vi "template-lstm-cell.vi"(7 "x":T1, 9 "h":T1, 11 "c":T1) -> (1 "h + 1":T1, 3 "c + 1":T1)   [LabVIEW 2020]
uses:
  <vilib>/Analysis/Matrix/Datatypes/RealMatrix.ctl
  <vilib>/Analysis/Matrix/Numeric/Multiply/Multiply - RM,RM.vi
  <vilib>/Analysis/Matrix/Numeric/Add/Add - RM,RM.vi
  <vilib>/Analysis/Matrix/NI_Matrix.lvlib
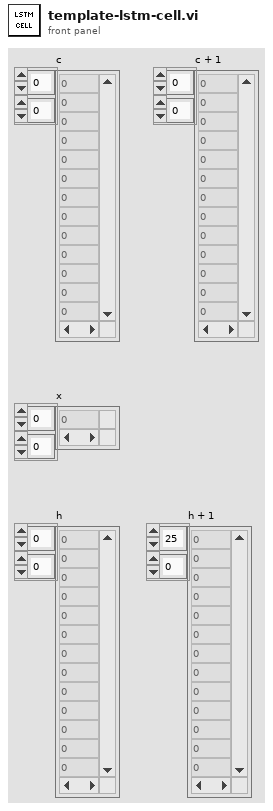
[diagram p1: front panel]
types:
  T1 = typedef "NI_Matrix.lvlib/RealMatrix.ctl" = dbl[][]
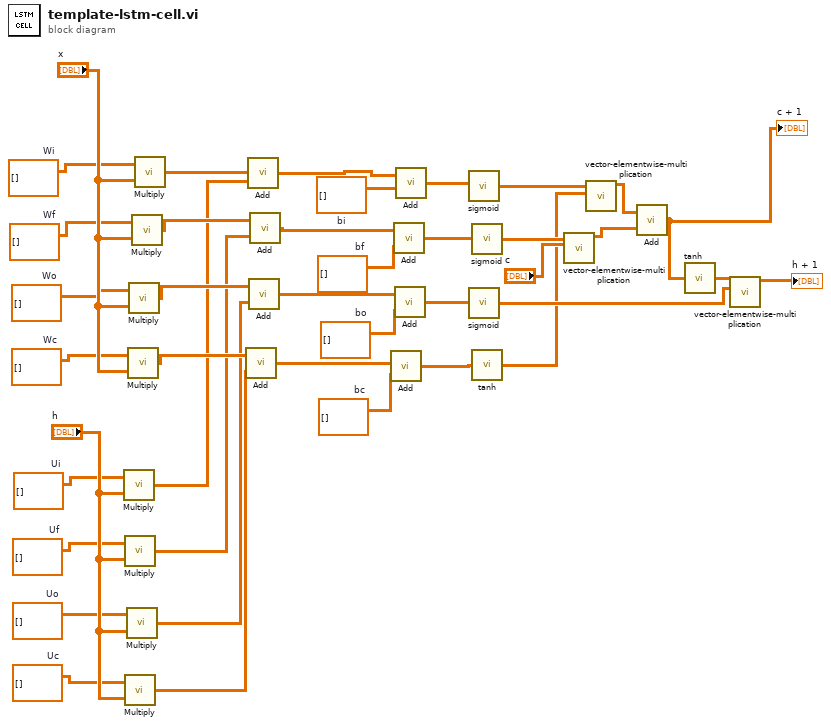
[diagram p0: block diagram]
diagram:
  w31 = T1 []  # Uo
  w17 = T1 []  # bo
  w38 = T1 []  # Wf
  w33 = T1 []  # Uf
  w37 = T1 []  # Wo
  w21 = T1 []  # bi
  w34 = T1 []  # Ui
  w39 = T1 []  # Wi
  w15 = T1 []  # bc
  w32 = T1 []  # Uc
  w36 = T1 []  # Wc
  w19 = T1 []  # bf
  n1 = call-poly <vilib>:"Multiply.vi"("Real Matrix B"="h", "Real Matrix A"=w34) -> ("A * B"=w26:T1)
  n2 = call-poly <vilib>:"Multiply.vi"("Real Matrix B"="h", "Real Matrix A"=w33) -> ("A * B"=w25:T1)
  n3 = call-poly <vilib>:"Multiply.vi"("Real Matrix B"="h", "Real Matrix A"=w32) -> ("A * B"=w23:T1)
  n4 = call-poly <vilib>:"Multiply.vi"("Real Matrix B"="h", "Real Matrix A"=w31) -> ("A * B"=w24:T1)
  n5 = call-poly <vilib>:"Multiply.vi"("Real Matrix B"="x", "Real Matrix A"=w36) -> ("A * B"=w27:T1)
  n6 = call-poly <vilib>:"Multiply.vi"("Real Matrix B"="x", "Real Matrix A"=w37) -> ("A * B"=w28:T1)
  n7 = call-poly <vilib>:"Multiply.vi"("Real Matrix B"="x", "Real Matrix A"=w38) -> ("A * B"=w29:T1)
  n8 = call-poly <vilib>:"Multiply.vi"("Real Matrix B"="x", "Real Matrix A"=w39) -> ("A * B"=w30:T1)
  n9 = call-poly <vilib>:"Add.vi"("Real Matrix B"=w23, "Real Matrix A"=w27) -> ("A + B"=w16:T1)
  n10 = call-poly <vilib>:"Add.vi"("Real Matrix B"=w26, "Real Matrix A"=w30) -> ("A + B"=w22:T1)
  n11 = call-poly <vilib>:"Add.vi"("Real Matrix B"=w24, "Real Matrix A"=w28) -> ("A + B"=w18:T1)
  n12 = call-poly <vilib>:"Add.vi"("Real Matrix B"=w25, "Real Matrix A"=w29) -> ("A + B"=w20:T1)
  n13 = call-poly <vilib>:"Add.vi"("Real Matrix B"=w15, "Real Matrix A"=w16) -> ("A + B"=w10:T1)
  n14 = call-poly <vilib>:"Add.vi"("Real Matrix B"=w19, "Real Matrix A"=w20) -> ("A + B"=w13:T1)
  n15 = call-poly <vilib>:"Add.vi"("Real Matrix B"=w17, "Real Matrix A"=w18) -> ("A + B"=w12:T1)
  n16 = call-poly <vilib>:"Add.vi"("Real Matrix B"=w21, "Real Matrix A"=w22) -> ("A + B"=w14:T1)
  n17 = call "sigmoid.vi"("x"=w14) -> ("y"=w4:T1)
  n18 = call "sigmoid.vi"("x"=w12) -> ("y"=w7:T1)
  n19 = call "sigmoid.vi"("x"=w13) -> ("y"=w9:T1)
  n20 = call "tanh.vi"("x"=w10) -> ("y"=w5:T1)
  n21 = call "vector-elementwise-multiplication.vi"("Matrix in"="c", "Matrix 1"=w9) -> ("elementwise product"=w2:T1)  [unwired: 9 in]
  n22 = call "vector-elementwise-multiplication.vi"("Matrix in"=w5, "Matrix 1"=w4) -> ("elementwise product"=w3:T1)  [unwired: 9 in]
  n23 = call-poly <vilib>:"Add.vi"("Real Matrix B"=w2, "Real Matrix A"=w3) -> ("A + B"=w1:T1)
  "c + 1" <- w1
  n24 = call "tanh.vi"("x"=w1) -> ("y"=w8:T1)
  n25 = call "vector-elementwise-multiplication.vi"("Matrix in"=w7, "Matrix 1"=w8) -> ("elementwise product"=→"h + 1":T1)  [unwired: 9 in]
